vi "Revision Query.vi"(0 "VISA resource name":refnum<visa-resource-name>, 5 "error in (no error)":errorcluster) -> (14 "VISA resource name out":refnum<visa-resource-name>, 17 "Instr Driver Revision":string, 18 "Instr Firmware Revision":string, 19 "error out":errorcluster)   [LabVIEW 2018, in "Keithley 2000.lvlib"]
doc: "This VI queries the current instrument firmware revision and instrument driver revision.\n\nThis Instrument Driver's Revision number is 2.0 and is compatible with Instrument Firmware Revision A13/A02.\n\nke2000\nCreated By: National Instruments (Adam Kemp)\nRelease Date: 11/03\nOriginally Developed in LabVIEW Version: 7.0\n\nModification History:\n\nREV 1.0, 01/1995\nOriginal Release.\n\nREV 2.0, 11/2003, LV 7.0\nCreated by: Adam Kemp, NI\nRewrote Driver to include major API updates and to make consistant with current instrument driver guidelines. Version 2.0 and above are not backward compatible with version 1.x\n\nREV 2.1, 10/2004, LV 7.0\nUpdated by: Matthew McClintock, NI\n- Configure an immeadiate trigger in the Default Instrument Setup VI\n- Reordered the sequence of commands in Wait for SRQ to avoid race conditions"
uses:
  <instrlib>/Keithley 2000/Keithley 2000.lvlib
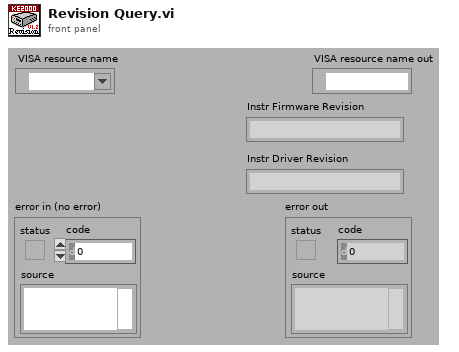
[diagram p1: front panel]
types:
  T1 = cluster{"Major":u16, "Minor":u16, "Fix":u16, "Build":u16}
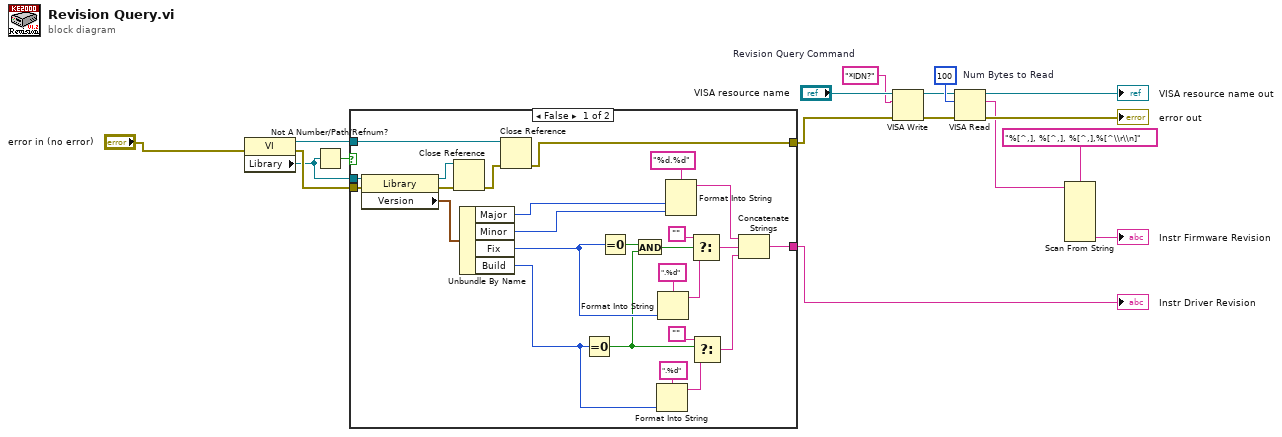
[diagram p0: block diagram]
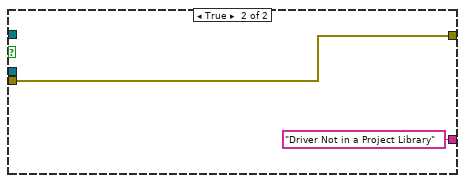
[diagram p2: hidden frame]
diagram:
  w10 = "*IDN?"  # Revision Query Command
  w13 = u32 100  # Num Bytes to Read
  n1 = property class="VI"(error in="error in (no error)") -> (reference out=w7:refnum<vi>, error out=w6:errorcluster, "Library"=w5:refnum<vi>)  [unwired: 1 in]
  n2 = Not A Number/Path/Refnum?(number/path/refnum=w5) -> (NaN/Path/Refnum?=w4:bool)
  n3 = case shown="False" w4 {
    tunnel: w7 -> [w40 _]
    tunnel: w6 -> [w25 w45]
    tunnel: [w20 w45] -> w1
    tunnel: [w19 "Driver Not in a Project Library"] -> w3
    tunnel: w5 -> [w18 _]
    frame False {
      n4 = property class="Library"(reference=w18, error in=w25) -> (reference out=w42:refnum<vi>, error out=w43:errorcluster, "Version"=w39:T1)
      n5 = Close Reference(reference=w42, error in (no error)=w43) -> (error out=w41:errorcluster)
      n6 = Unbundle By Name(w39) -> ("Major"=w28:u16, "Minor"=w27:u16, "Fix"=w24:u16, "Build"=w26:u16)
      n7 = Close Reference(reference=w40, error in (no error)=w41) -> (error out=w20:errorcluster)
      n8 = Equal To 0?(x=w26) -> (x = 0?=w22:bool)
      n9 = Equal To 0?(x=w24) -> (x = 0?=w23:bool)
      n10 = And(x=w23, y=w22) -> (x .and. y?=w21:bool)
      n11 = Format Into String(format string=".%d", w26) -> (resulting string=w32:string)  [unwired: 2 in, 1 out]
      n12 = Format Into String(format string=".%d", w24) -> (resulting string=w36:string)  [unwired: 2 in, 1 out]
      n13 = Format Into String(format string="%d.%d", w28, w27) -> (resulting string=w34:string)  [unwired: 2 in, 1 out]
      n14 = Select(t="", s=w21, f=w36) -> (s? t:f=w33:string)
      n15 = Select(t="", s=w22, f=w32) -> (s? t:f=w29:string)
      n16 = Concatenate Strings(w34, w33, w29) -> (w19:string)
    }
    frame True {
    }
  }
  "Instr Driver Revision" <- w3
  n17 = VISA Write(VISA resource name="VISA resource name", write buffer=w10, error in (no error)=w1) -> (VISA resource name out=w12:refnum<visa-resource-name>, error out=w11:errorcluster)  [unwired: 1 out]
  n18 = VISA Read(VISA resource name=w12, byte count=w13, error in (no error)=w11) -> (VISA resource name out=→"VISA resource name out":refnum<visa-resource-name>, read buffer=w9:string, error out=→"error out":errorcluster)  [unwired: 1 out]
  n19 = Scan From String(format string="%[^,], %[^,], %[^,],%[^\\r\\n]", input string=w9) -> (output 4=→"Instr Firmware Revision":string)  [unwired: 9 in, 3 out]
